vi "Main.vi"(11 "Module Admin":refnum<class "Delacor_lib_QMH_Cloneable Module Admin.lvclass">) -> ()   [LabVIEW 2015, in "LV-WinSCP.lvlib"]
doc: "This template is based off of the Queued Message Handler design pattern and the Queued Message Handler project template that ships with LabVIEW.\n\nThe main difference is that the queue is private to this module and communication between modules is performed via Broadcast and Request events.\n\nRequest events are wrapped in public API methods and are handled in the Event Handling Loop (EHL) of this VI. Any module can register for Broadcast events sent by this module. The EHL generates messages based on user interface actions.\n\nThe Message Handling Loop (MHL) processes messages generated by the EHL, or by other messages. The messages are string values, so new messages can be added easily to the Message Cases case structure in the MHL. Each message cluster can also provide an optional value for Message Data, which is a variant that can be converted to whatever message-specific data is required.\n_____\nBased on DQMH Project Template 6.1.0.94."
uses:
  LV-WinSCP.lvlib
  <vilib>/Delacor/Delacor QMH/Libraries/Message Queue_class/Delacor_lib_QMH_Message Queue.lvclass
  Module Data--cluster.ctl
  <vilib>/Utility/miscctls.llb/LVPointTypeDef.ctl
  <vilib>/Utility/error.llb/Error Cluster From Error Code.vi
  <vilib>/ErrorRing/Error Ring.xnode
  <vilib>/Delacor/Delacor QMH/Libraries/Message Queue_class/Delacor_lib_QMH_Enqueue Message (Single).vi
  Stop Argument--cluster.ctl
  <vilib>/Delacor/Delacor QMH/Libraries/Cloneable Module Admin_class/Delacor_lib_QMH_Cloneable Module Admin.lvclass
  Initialize Session (Reply Payload)--cluster.ctl
  Classes/SessionOptions/SessionOptions.lvclass
  Initialize Session Argument--cluster.ctl
  C:/Program Files (x86)/WinSCP/WinSCPnet.dll
  Program Files (x86)/WinSCP/WinSCPnet.dll
panel:
  out "error out":errorcluster
  out "Status":string
  in  "Simulate EHL Error":bool
  in  "Simulate MHL Error":bool
  # "Other QMH Modules communicate with this Module via its Public API (wrappers for its Request Events).\n\nThis Module communicates with other Modules via its Broadcast Events.\nAny module that wants to get these messages, just registers for this module's Broadcast events."
  # "This template is for the Delacor Modified Queued Message Handler design pattern.\n\nSee the block diagram for more information on how to use this template."
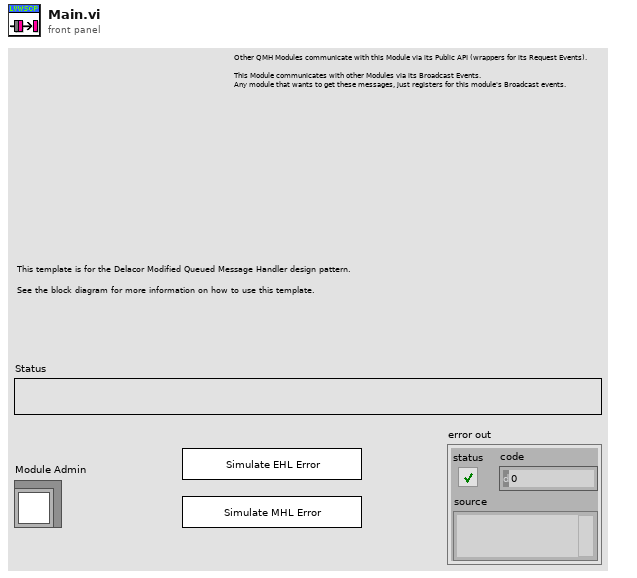
[diagram p1: front panel]
types:
  T1 = typedef "LV-WinSCP.lvlib/Request Events--cluster.ctl" = cluster{"Stop Module":refnum<user-event>, "Show Panel":refnum<user-event>, "Hide Panel":refnum<user-event>, "Show Diagram":refnum<user-event>, "Get Module Execution Status":refnum<user-event>, "Initialize Session":refnum<user-event>}
  T2 = typedef "LV-WinSCP.lvlib/Module Data--cluster.ctl" = cluster{"Status":string}
  T3 = enum32{"invalid lock state", "Not Locked", "Locked (No Password)", "Password-protected"}
  T4 = typedef "LV-WinSCP.lvlib/Stop Argument--cluster.ctl" = cluster{"Module ID":i32, "Origin":string, "Exit via Stop Module Req?":bool, "Wait for Module to stop?":bool}
  T5 = typedef "LV-WinSCP.lvlib/Initialize Session Argument--cluster.ctl" = cluster{"Module ID":i32, "SessionOptions":refnum<class "SessionOptions.lvclass">, "Wait Notifier":refnum<notifier>, "wait for reply":bool}
  T6 = typedef "LVPointTypeDef.ctl" = cluster{"Horizontal":i16, "Vertical":i16}
  T7 = enum32{"Invalid", "Standard", "Closed", "Hidden", "Minimized", "Maximized"}
  T8 = typedef "LV-WinSCP.lvlib/Initialize Session (Reply Payload)--cluster.ctl" = cluster{"Connected?":bool, "error":errorcluster}
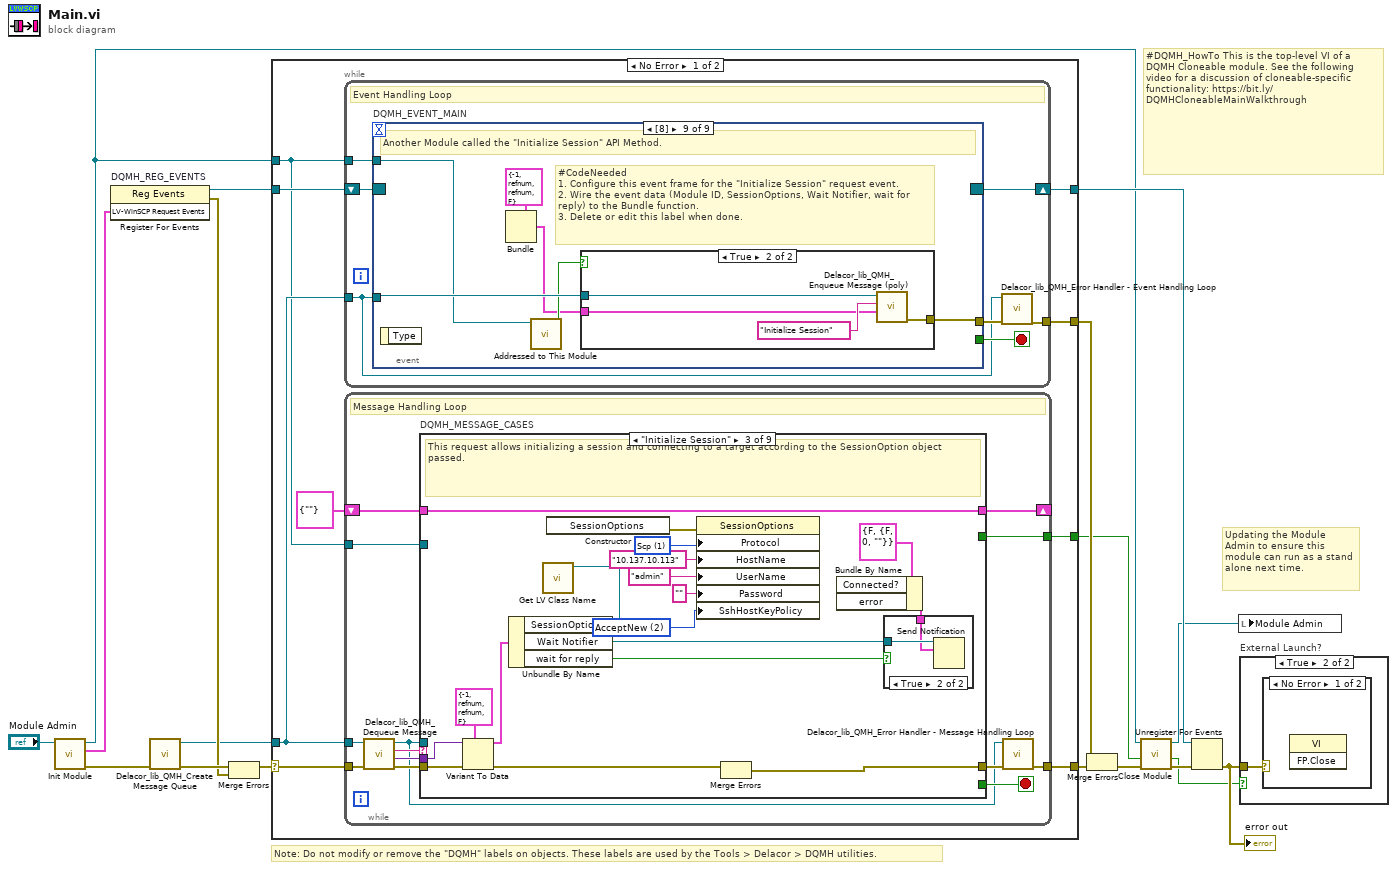
[diagram p0: block diagram]
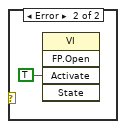
[diagram p3: hidden frame]
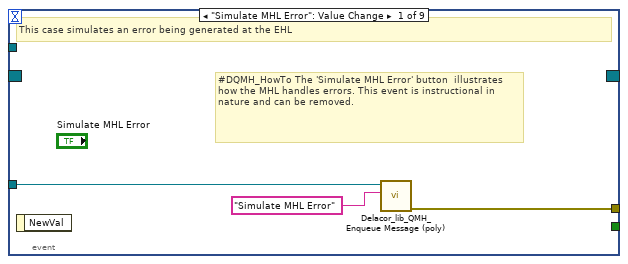
[diagram p4: hidden frame]
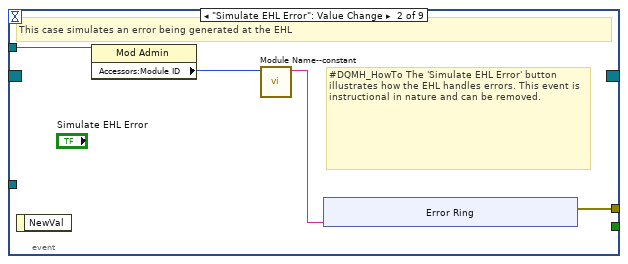
[diagram p5: hidden frame]
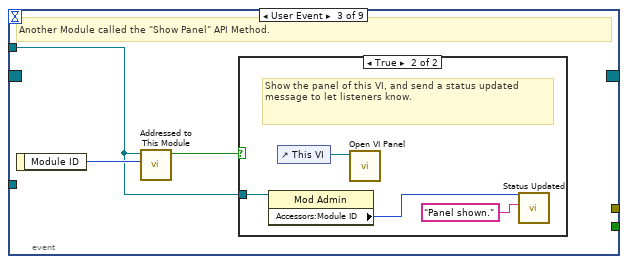
[diagram p6: hidden frame]
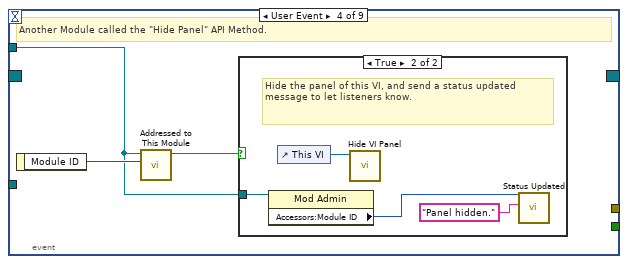
[diagram p8: hidden frame]
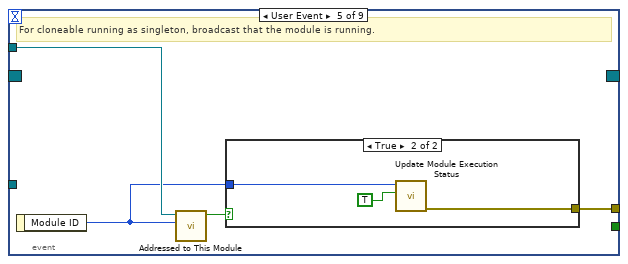
[diagram p10: hidden frame]
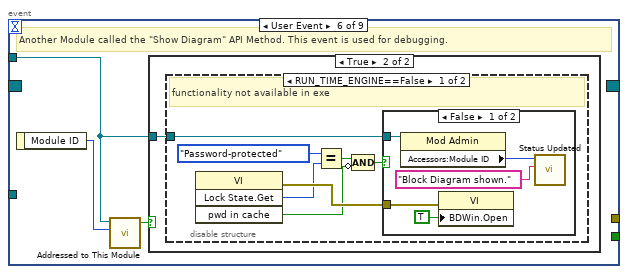
[diagram p12: hidden frame]
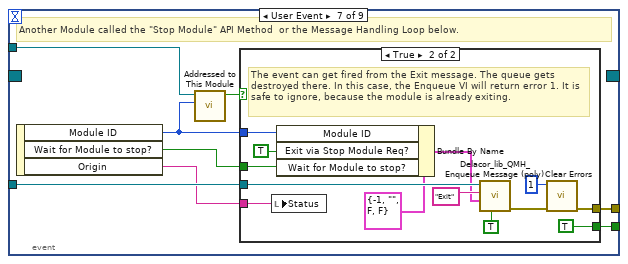
[diagram p16: hidden frame]
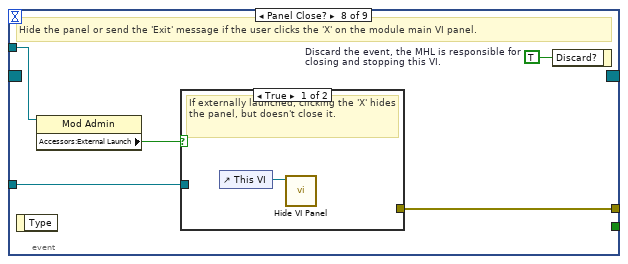
[diagram p18: hidden frame]
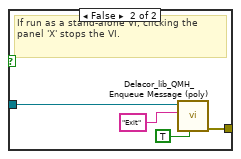
[diagram p19: hidden frame]
diagram:
  # "#DQMH_HowTo This is the top-level VI of a DQMH Cloneable module. See the following video for a discussion of cloneable-specific functionality: https://bit.ly/DQMHCloneableMainWalkthrough"
  # "Note: Do not modify or remove the \"DQMH\" labels on objects. These labels are used by the Tools > Delacor > DQMH utilities."
  # "Updating the Module Admin to ensure this module can run as a stand alone next time."
  n1 = call "Init Module.vi"("Cloneable Module Admin in"="Module Admin") -> ("error out"=w15:errorcluster, "LV-WinSCP Request Events"=w7:T1, "Cloneable Module Admin out"=w4:refnum<class "Delacor_lib_QMH_Cloneable Module Admin.lvclass">)  [unwired: 8 in]
  n2 = register-events "DQMH_REG_EVENTS"(w7) -> (reference out=w8:refnum<event-registration>, error out=w10:errorcluster)  [unwired: 2 in]
  n3 = call <vilib>:"Delacor_lib_QMH_Create Message Queue.vi"("error in"=w15) -> ("error out"=w12:errorcluster, "Message Queue"=w6:refnum<class "Delacor_lib_QMH_Message Queue.lvclass">)  [unwired: 9 in]
  n4 = Merge Errors(w12, w10) -> (w11:errorcluster)
  n5 = case shown="No Error" w11 {
    selector: w11 -> [w25 w253]
    tunnel: [w27 w252] -> w16
    tunnel: [w24 w260] -> w9
    tunnel: w8 -> [w22 w260]
    tunnel: w6 -> [w21 w251]
    tunnel: [w26 _] -> w17
    tunnel: w4 -> [w20 w256]
    tunnel: [w19 _] -> w2
    frame No Error {
      n6 = while {
        tunnel: w21 -> [w28]
        shift-right: [w31] -> w24
        shift-left: w22 -> [w32]
        tunnel: [w33] -> w26
        tunnel: w20 -> [w29]
        stop <- w30 stop-if-true
        # "Event Handling Loop"
        n7 = event "DQMH_EVENT_MAIN" shown="[8]" {
          selector: w32 -> [_ _ _ _ _ _ _ _ _]
          dyn-events: [_ _ _ _ _ _ _ _ _] -> w31
          timeout: _ -> [_ _ _ _ _ _ _ _ _]
          tunnel: [_ _ _ _ _ _ w89 _ _] -> w30
          tunnel: w28 -> [w36 _ _ _ _ _ w92 w108 w122]
          tunnel: [w37 w41 _ _ w66 _ w93 w111 w117] -> w34
          tunnel: w29 -> [_ w40 w49 w56 w64 w70 w91 w109 w120]
          event "Simulate MHL Error": Value Change {
            # "#DQMH_HowTo The 'Simulate MHL Error' button  illustrates how the MHL handles errors. This event is instructional in nature and can be removed."
            # "This case simulates an error being generated at the EHL"
            n8 = event-data() -> ()  [unwired: 1 in, 1 out]
            n9 = call-poly <vilib>:"Delacor_lib_QMH_Enqueue Message (poly).vi"("Message"="Simulate MHL Error", "Message Queue in"=w36) -> ("error out"=w37:errorcluster)  [unwired: 8 in, 1 out]
          }
          event "Simulate EHL Error": Value Change {
            # "#DQMH_HowTo The 'Simulate EHL Error' button  illustrates how the EHL handles errors. This event is instructional in nature and can be removed."
            # "This case simulates an error being generated at the EHL"
            n10 = event-data() -> ()  [unwired: 1 in, 1 out]
            n11 = property class="Mod Admin"(reference=w40) -> ("Accessors:Module ID"=w39:i32)  [unwired: 1 in, 2 out]
            n12 = call "Module Name--constant.vi"("Module ID"=w39) -> ("Module Name"=w38:string)  [unwired: 10 in]
            n13 = xnode "Error Ring"("parameter 0"=w38) -> ("error out"=w41:errorcluster)
          }
          event User Event {
            # "Another Module called the \"Show Panel\" API Method."
            n14 = event-data() -> ("Module ID"=w50:i32)  [unwired: 1 in]
            n15 = call "Addressed to This Module.vi"("Module ID from Argument"=w50, "Module Admin"=w49) -> ("Addressed to this instance?"=w51:bool)  [unwired: 8 in, 1 out]
            n16 = case shown="True" w51 {
              tunnel: w49 -> [_ w53]
              frame False {
              }
              frame True {
                # "Show the panel of this VI, and send a status updated message to let listeners know."
                n17 = property class="Mod Admin"(reference=w53) -> ("Accessors:Module ID"=w52:i32)  [unwired: 1 in, 2 out]
                n18 = control-ref of="This VI"() -> (w55:refnum<vi>)
                n19 = call "Open VI Panel.vi"("VI"=w55) -> ()  [unwired: 10 in, 1 out]
                n20 = call "Status Updated.vi"("Status"="Panel shown." ("format string"), "Module ID"=w52) -> ()  [unwired: 9 in, 1 out]
              }
            }
          }
          event User Event {
            # "Another Module called the \"Hide Panel\" API Method."
            n21 = event-data() -> ("Module ID"=w57:i32)  [unwired: 1 in]
            n22 = call "Addressed to This Module.vi"("Module ID from Argument"=w57, "Module Admin"=w56) -> ("Addressed to this instance?"=w58:bool)  [unwired: 8 in, 1 out]
            n23 = case shown="True" w58 {
              tunnel: w56 -> [_ w60]
              frame False {
              }
              frame True {
                # "Hide the panel of this VI, and send a status updated message to let listeners know."
                n24 = property class="Mod Admin"(reference=w60) -> ("Accessors:Module ID"=w59:i32)  [unwired: 1 in, 2 out]
                n25 = control-ref of="This VI"() -> (w62:refnum<vi>)
                n26 = call "Hide VI Panel.vi"("VI"=w62) -> ()  [unwired: 10 in, 1 out]
                n27 = call "Status Updated.vi"("Status"="Panel hidden." ("format string"), "Module ID"=w59) -> ()  [unwired: 9 in, 1 out]
              }
            }
          }
          event User Event {
            # "For cloneable running as singleton, broadcast that the module is running."
            n28 = event-data() -> ("Module ID"=w63:i32)  [unwired: 1 in]
            n29 = call "Addressed to This Module.vi"("Module ID from Argument"=w63, "Module Admin"=w64) -> ("Addressed to this instance?"=w65:bool)  [unwired: 8 in, 1 out]
            n30 = case shown="True" w65 {
              tunnel: [_ w69] -> w66
              tunnel: w63 -> [_ w68]
              frame False {
              }
              frame True {
                n31 = call "Update Module Execution Status.vi"("Running?"=TRUE, "Module ID"=w68) -> ("error out"=w69:errorcluster)  [unwired: 9 in]
              }
            }
          }
          event User Event {
            # "Another Module called the \"Show Diagram\" API Method. This event is used for debugging."
            n32 = event-data() -> ("Module ID"=w71:i32)  [unwired: 1 in]
            n33 = call "Addressed to This Module.vi"("Module ID from Argument"=w71, "Module Admin"=w70) -> ("Addressed to this instance?"=w72:bool)  [unwired: 8 in, 1 out]
            n34 = case shown="True" w72 {
              tunnel: w70 -> [_ w73]
              frame False {
              }
              frame True {
                n35 = disable-structure shown="RUN_TIME_ENGINE==False" {
                  disable-tunnel: w73 -> [w74 _]
                  frame condition #0 (active) {
                    # "functionality not available in exe"
                    n36 = invoke class="VI" method="Lock State.Get"() -> (error out=w80:errorcluster, "Get Lock State"=w79:T3, "pwd in cache"=w76:bool)  [unwired: 4 in, 1 out]
                    n37 = Equal?(x=T3."Password-protected", y=w79) -> (x = y?=w77:bool)
                    n38 = Compound Arithmetic op=AND(w77, invert w76) -> (w75:bool)
                    n39 = case shown="False" w75 {
                      tunnel: w80 -> [w85 _]
                      tunnel: w74 -> [w82 _]
                      frame False {
                        n40 = property class="Mod Admin"(reference=w82) -> ("Accessors:Module ID"=w81:i32)  [unwired: 1 in, 2 out]
                        n41 = property class="VI"(error in=w85, "BDWin.Open"=TRUE ("Block Diagram Window:Open")) -> ()  [unwired: 1 in, 2 out]
                        n42 = call "Status Updated.vi"("Status"="Block Diagram shown." ("format string"), "Module ID"=w81) -> ()  [unwired: 9 in, 1 out]
                      }
                      frame True {
                        # "Password-protected VI, and the password is not in the cache. Do not show the diagram."
                      }
                    }
                  }
                  frame condition #1 {
                  }
                }
              }
            }
          }
          event User Event {
            # "Another Module called the \"Stop Module\" API Method  or the Message Handling Loop below."
            n43 = event-data() -> ("Module ID"=w87:i32, "Wait for Module to stop?"=w88:bool, "Origin"=w86:string)  [unwired: 1 in]
            n44 = call "Addressed to This Module.vi"("Module ID from Argument"=w87, "Module Admin"=w91) -> ("Addressed to this instance?"=w90:bool)  [unwired: 8 in, 1 out]
            n45 = case shown="True" w90 {
              tunnel: [_ w105] -> w93
              tunnel: w92 -> [_ w101]
              tunnel: [_ TRUE] -> w89
              tunnel: w88 -> [_ w96]
              tunnel: w87 -> [_ w98]
              tunnel: w86 -> [_ w94]
              frame False {
              }
              frame True {
                # "The event can get fired from the Exit message. The queue gets destroyed there. In this case, the Enqueue VI will return error 1. It is safe to ignore, because the module is already exiting."
                n46 = local write "Status"(w94) -> ()
                n47 = Bundle By Name(cluster=T4 {"Module ID"=-1, "Origin"="", "Exit via Stop Module Req?"=FALSE, "Wait for Module to stop?"=FALSE} ("Stop Argument"), "Module ID"=w98, "Exit via Stop Module Req?"=TRUE, "Wait for Module to stop?"=w96) -> (w95:T4)
                n48 = call-poly <vilib>:"Delacor_lib_QMH_Enqueue Message (poly).vi"("Priority Message? (F)"=TRUE, "Message Data"=w95, "Message"="Exit", "Message Queue in"=w101) -> ("error out"=w106:errorcluster)  [unwired: 6 in, 1 out]
                n49 = call <vilib>:"Clear Errors.vi"("error in (no error)"=w106, "specific error code to clear (0: all)"=1) -> ("error out"=w105:errorcluster)  [unwired: 4 in, 1 out]
              }
            }
          }
          event Panel Close? {
            w110 = TRUE  # Discard the event, the MHL is responsible for closing and stopping this VI.
            # "Hide the panel or send the 'Exit' message if the user clicks the 'X' on the module main VI panel."
            n50 = event-data() -> ()  [unwired: 1 in, 1 out]
            n51 = property class="Mod Admin"(reference=w109) -> ("Accessors:External Launch"=w107:bool)  [unwired: 1 in, 2 out]
            n52 = case shown="True" w107 {
              tunnel: w108 -> [_ w115]
              tunnel: [_ w116] -> w111
              frame True {
                # "If externally launched, clicking the 'X' hides the panel, but doesn't close it."
                n53 = control-ref of="This VI"() -> (w112:refnum<vi>)
                n54 = call "Hide VI Panel.vi"("VI"=w112) -> ()  [unwired: 10 in, 1 out]
              }
              frame False {
                # "If run as a stand-alone VI, clicking the panel 'X' stops the VI."
                n55 = call-poly <vilib>:"Delacor_lib_QMH_Enqueue Message (poly).vi"("Priority Message? (F)"=TRUE, "Message"="Exit", "Message Queue in"=w115) -> ("error out"=w116:errorcluster)  [unwired: 7 in, 1 out]
              }
            }
            n56 = event-data("Discard?"=w110) -> ()  [unwired: 1 in, 1 out]
          }
          event #8 (no event record) {
            # "#CodeNeeded\n1. Configure this event frame for the \"Initialize Session\" request event.\n2. Wire the event data (Module ID, SessionOptions, Wait Notifier, wait for reply) to the Bundle function.\n3. Delete or edit this label when done."
            # "Another Module called the \"Initialize Session\" API Method."
            n57 = event-data() -> ()  [unwired: 1 in, 1 out]
            n58 = Bundle(cluster=T5 {"Module ID"=-1, "SessionOptions"=refnum, "Wait Notifier"=refnum, "wait for reply"=FALSE} ("Initialize Session Argument")) -> (w118:T5)  [unwired: 4 in]
            n59 = call "Addressed to This Module.vi"("Module Admin"=w120) -> ("Addressed to this instance?"=w121:bool)  [unwired: 9 in, 1 out]
            n60 = case shown="True" w121 {
              tunnel: w122 -> [_ w126]
              tunnel: w118 -> [_ w124]
              tunnel: [_ w123] -> w117
              frame False {
              }
              frame True {
                n61 = call-poly <vilib>:"Delacor_lib_QMH_Enqueue Message (poly).vi"("Message Data"=w124, "Message"="Initialize Session", "Message Queue in"=w126) -> ("error out"=w123:errorcluster)  [unwired: 7 in, 1 out]
              }
            }
          }
        }
        n62 = call-dynamic "Delacor_lib_QMH_Error Handler - Event Handling Loop.vi"("error in"=w34, "Message Queue in"=w28) -> ("dup error in"=w33:errorcluster)  [unwired: 8 in, 1 out]
      }
      n63 = while {
        tunnel: w21 -> [w130]
        shift-right: [w134] -> _
        shift-left: T2 {"Status"=""} ("Data Cluster") -> [w135]
        tunnel: w25 -> [w138]
        tunnel: [w136] -> w27
        tunnel: w20 -> [w128]
        tunnel: [w127] -> w19
        stop <- w133 stop-if-true
        # "Message Handling Loop"
        n64 = call-dynamic "Delacor_lib_QMH_Dequeue Message.vi"("error in"=w138, "Message Queue in"=w130) -> ("error out"=w137:errorcluster, "Message Data"=w131:variant, "Message"=w132:string, "Message Queue out"=w129:refnum<class "Delacor_lib_QMH_Message Queue.lvclass">)  [unwired: 6 in]
        n65 = case "DQMH_MESSAGE_CASES" shown="\"Initialize Session\"" w132 {
          selector: w132 -> [_ _ _ _ _ _ _ _ w238]
          tunnel: w129 -> [_ _ _ _ _ w189 _ w228 _]
          tunnel: w137 -> [w158 w162 w180 w185 w187 w198 w211 w234 w240]
          tunnel: [w156 w162 w170 w184 w187 w194 w210 w231 w241] -> w139
          tunnel: w135 -> [w149 w161 w179 w183 w186 w193 w208 w227 w239]
          tunnel: [w148 w161 w179 w183 w186 w193 w208 w227 w239] -> w134
          tunnel: [_ _ _ _ _ _ _ w226 _] -> w133
          tunnel: w131 -> [_ _ w177 _ _ w192 _ w224 _]
          tunnel: w128 -> [w143 _ _ _ _ w191 w206 w220 w236]
          tunnel: [_ _ _ _ _ _ _ w222 _] -> w127
          frame "Initialize" {
            w140 = "Initial Message" ("Initial Message")
            # "#CodeNeeded - Initialize the appearance of the front panel."
            # "#CodeNeeded - Initialize your state data here."
            # "Initialize - Any operation that needs to be done before the module can receive messages. Synchronize Caller Events.vi will inform Start Module.vi that the module has launched and is ready to receive messages. Module Did Init.vi will broadcast that the module initialized."
            n66 = call "Synchronize Caller Events.vi"("error in (no error)"=w158, "Module Admin"=w143) -> ("error out"=w157:errorcluster, "Module Admin out"=w142:refnum<class "Delacor_lib_QMH_Cloneable Module Admin.lvclass">)  [unwired: 8 in]
            n67 = property class="Mod Admin"(reference=w142) -> ("Accessors:Module ID"=w145:i32, "Accessors:External Launch"=w144:bool)  [unwired: 1 in, 2 out]
            n68 = call "Module Name--constant.vi"("Module ID"=w145) -> ("Module Name"=w153:string)  [unwired: 10 in]
            n69 = property class="VI"("Front Panel.Title"=w153) -> (reference out=w155:refnum<vi>, error out=w160:errorcluster)  [unwired: 2 in]
            n70 = Select(t=T7."Hidden" ("State"), s=w144, f=T7."Standard" ("State")) -> (s? t:f=w150:T7)
            n71 = invoke class="VI" method="FP.Open"(reference=w155, error in=w160, "State"=w150) -> (reference out=w154:refnum<vi>, error out=w159:errorcluster)  [unwired: 2 in, 3 out]
            n72 = call "Module Name--constant.vi"("Module ID"=w145) -> ("Module Name"=w146:string)  [unwired: 10 in]
            n73 = Bundle By Name(cluster=w149, "Status"=w140) -> (w148:T2)
            n74 = invoke class="VI" method="FP.Center"(reference=w154, error in=w159) -> ()  [unwired: 1 in, 3 out]
            n75 = property on="Pane" class="Pane"("Origin"=T6 {"Horizontal"=0, "Vertical"=0}) -> ()  [unwired: 2 in, 2 out]
            n76 = call "Module Did Init.vi"("error in (no error)"=w157, "Initialized?"=TRUE, "Origin"=w146, "Module ID"=w145) -> ("error out"=w156:errorcluster)  [unwired: 7 in]
            "Status" <- w140
          }
          frame "---Module Specific---" {
            # "Separator -- The following cases handle messages specific to this Module."
          }
          frame "Initialize Session" {
            w166 = 2 items=["Check", "GiveUpSecurityAndAcceptAny", "AcceptNew"] ("SshHostKeyPolicy")
            w167 = 1 items=["Sftp", "Scp", "Ftp", "Webdav", "S3"] ("Protocol")
            # "This request allows initializing a session and connecting to a target according to the SessionOption object passed."
            n77 = Variant To Data(error in=w180, type=T5 {"Module ID"=-1, "SessionOptions"=refnum, "Wait Notifier"=refnum, "wait for reply"=FALSE} ("Initialize Session Argument"), Variant=w177) -> (data=w175:T5, error out=w178:errorcluster)
            n78 = Unbundle By Name(w175) -> ("SessionOptions"=w169:refnum<class "SessionOptions.lvclass">, "Wait Notifier"=w174:refnum<notifier>, "wait for reply"=w173:bool)
            n79 = call <vilib>:"Get LV Class Name.vi"("object"=w169) -> ()  [unwired: 9 in, 2 out]
            n80 = constructor class="SessionOptions"() -> (error out=w168:errorcluster)  [unwired: 3 in, 2 out]
            n81 = property class="SessionOptions"(error in=w168, "Protocol"=w167, "HostName"="10.137.10.113", "UserName"="admin", "Password"="", "SshHostKeyPolicy"=w166) -> ()  [unwired: 1 in, 2 out]
            n82 = Merge Errors(w178) -> (w170:errorcluster)  [unwired: 1 in]
            n83 = Bundle By Name(cluster=T8 {"Connected?"=FALSE, "error"={"status"=FALSE, "code"=0, "source"=""}} ("Initialize Session (Reply Payload)")) -> (w172:T8)  [unwired: 2 in]
            n84 = case shown="True" w173 {
              tunnel: w174 -> [_ w182]
              tunnel: w172 -> [_ w181]
              frame False {
              }
              frame True {
                n85 = Send Notification(notification=w181, notifier=w182) -> ()  [unwired: 1 in, 2 out]
              }
            }
          }
          frame "---Copy This Frame---" {
            # "Duplicate this frame when creating new messages.  Change this comment in the duplicated frame to describe this message."
            n86 = Merge Errors(w185) -> (w184:errorcluster)
          }
          frame "---Exit and Error Handling---" {
            # "Separator - the following cases handle errors and exit messages."
          }
          frame "Error" {
            # "#CodeRecommended - If you ever change the name of this \"Error\" message, you'll need to update the name in the Check Loop Error.vi as well."
            # "#CodeRecommended - If the module is running in standalone mode (External Launch = FALSE), this code will pop up an error dialog and call the 'Exit' message if an error occurs. Add more fine-grained error handling here."
            # "Error - Check the error message data and respond accordingly. This message is sent by the \"Error Handler\" VIs at the end of each loop in this application."
            n87 = property class="Mod Admin"(reference=w191) -> ("Accessors:External Launch"=w190:bool, "Accessors:Module ID"=w188:i32)  [unwired: 1 in, 2 out]
            n88 = Variant To Data(error in=w198, type=errorcluster {"status"=FALSE, "code"=0, "source"=""} ("error constant"), Variant=w192) -> (data=w199:errorcluster, error out=w196:errorcluster)
            n89 = call "Error Reported.vi"("Error"=w199, "Module ID"=w188) -> ()  [unwired: 9 in, 1 out]
            n90 = case shown="False" w190 {
              tunnel: [w204 _] -> w195
              tunnel: w189 -> [w202 _]
              tunnel: w199 -> [w203 _]
              frame False {
                # "If the module is running standalone, then pop up an error dialog and call the \"Exit\" message."
                n91 = call <vilib>:"Simple Error Handler.vi"("error in (no error)"=w203) -> ()  [unwired: 4 in, 5 out]
                n92 = call-poly <vilib>:"Delacor_lib_QMH_Enqueue Message (poly).vi"("Priority Message? (F)"=TRUE, "Message"="Exit", "Message Queue in"=w202) -> ("error out"=w204:errorcluster)  [unwired: 7 in, 1 out]
              }
              frame True {
                # "If the module was launched externally, calling the Error Reported broadcast VI is the only action performed by the \"Error\" message. The module's caller can then process the error appropriately."
              }
            }
            n93 = Merge Errors(w196, w195) -> (w194:errorcluster)
            n94 = local write "error out"(w194) -> ()
          }
          frame "Simulate MHL Error" {
            # "#DQMH_HowTo The 'Simulate MHL Error' button  illustrates how the MHL handles errors. This event is instructional in nature and can be removed."
            # "Simulate an error occurring at the MHL"
            n95 = property class="Mod Admin"(reference=w206) -> ("Accessors:Module ID"=w207:i32)  [unwired: 1 in, 2 out]
            n96 = call "Module Name--constant.vi"("Module ID"=w207) -> ("Module Name"=w205:string)  [unwired: 10 in]
            n97 = xnode "Error Ring"("parameter 0"=w205) -> ("error out"=w209:errorcluster)
            n98 = Merge Errors(w211, w209) -> (w210:errorcluster)
          }
          frame "Exit" {
            w225 = 91  # 91: not all Exit messages will have an argument
            w226 = TRUE  # Stop the VI
            # "Release the message queue reference"
            # "#CodeNeeded - Add any required cleanup code here."
            # "Exit - Exit the application."
            n99 = Variant To Data(error in=w234, type=T4 {"Module ID"=-1, "Origin"="", "Exit via Stop Module Req?"=FALSE, "Wait for Module to stop?"=FALSE} ("Stop Argument"), Variant=w224) -> (data=w221:T4, error out=w229:errorcluster)
            n100 = call <vilib>:"Clear Errors.vi"("error in (no error)"=w229, "specific error code to clear (0: all)"=w225) -> ("error out"=w233:errorcluster)  [unwired: 4 in, 1 out]
            n101 = control-ref of="This VI"() -> (w219:refnum<vi>)
            n102 = call-dynamic "Delacor_lib_QMH_Release Message Queue.vi"("error in"=w233, "Message Queue"=w228) -> ("error out"=w232:errorcluster)  [unwired: 9 in]
            n103 = call "Handle Exit.vi"("Stop Argument"=w221, "Module Admin in"=w220, "VI reference"=w219) -> ("error out"=w230:errorcluster, "Wait for Stop?"=w222:bool)  [unwired: 7 in]
            n104 = Merge Errors(w232, w230) -> (w231:errorcluster)
          }
          frame Default {
            # "'Default' case only runs if there is a message that isn't defined in any of the other cases.  Output a programming error."
            n105 = property class="Mod Admin"(reference=w236) -> ("Accessors:Module ID"=w235:i32)  [unwired: 1 in, 2 out]
            n106 = call "Module Name--constant.vi"("Module ID"=w235) -> ("Module Name"=w237:string)  [unwired: 10 in]
            n107 = xnode "Error Ring"("parameter 0"=w238, "parameter 1"=w237) -> ("error out"=w242:errorcluster)
            n108 = Merge Errors(w240, w242) -> (w241:errorcluster)
          }
        }
        n109 = call-dynamic "Delacor_lib_QMH_Error Handler - Message Handling Loop.vi"("error in"=w139, "Message Queue in"=w129) -> ("dup error in"=w136:errorcluster)  [unwired: 8 in, 1 out]
      }
    }
    frame Error {
      n110 = call "Synchronize Caller Events.vi"("Module Admin"=w256) -> ("Module Admin out"=w255:refnum<class "Delacor_lib_QMH_Cloneable Module Admin.lvclass">)  [unwired: 9 in, 1 out]
      n111 = property class="Mod Admin"(reference=w255) -> ("Accessors:Module ID"=w254:i32)  [unwired: 1 in, 2 out]
      n112 = call-dynamic "Delacor_lib_QMH_Release Message Queue.vi"("error in"=w253, "Message Queue"=w251) -> ("error out"=w252:errorcluster)  [unwired: 9 in]
      n113 = call "Module Name--constant.vi"("Module ID"=w254) -> ("Module Name"=w259:string)  [unwired: 10 in]
      n114 = Format Into String(format string="An error occurred during initialization. %s is no longer running.", w259) -> (resulting string=w257:string)  [unwired: 2 in, 1 out]
      n115 = call "Error Reported.vi"("Additional Information"=w257, "Error"=w252, "Module ID"=w254) -> ()  [unwired: 8 in, 1 out]
    }
  }
  n116 = Merge Errors(w17, w16) -> (w18:errorcluster)
  n117 = call "Close Module.vi"("error in"=w18, "Wait for stop?"=w2, "Module Admin in"=w4) -> ("error out"=w14:errorcluster, "External Launch"=w1:bool, "Module Admin out"=w3:refnum<class "Delacor_lib_QMH_Cloneable Module Admin.lvclass">)  [unwired: 6 in]
  n118 = Unregister For Events(event registration refnum=w9, error in=w14) -> (error out=w13:errorcluster)
  "error out" <- w13
  n119 = local write "Module Admin"(w3) -> ()
  n120 = case "External Launch?" shown="True" w1 {
    tunnel: w13 -> [_ w261]
    frame False {
    }
    frame True {
      n121 = case shown="No Error" w261 {
        frame No Error {
          n122 = invoke class="VI" method="FP.Close"() -> ()  [unwired: 3 in, 3 out]
        }
        frame Error {
          n123 = invoke class="VI" method="FP.Open"("Activate"=TRUE ("Activate?")) -> ()  [unwired: 4 in, 5 out]
        }
      }
    }
  }
